vi "Set Colour.vi"(0 "Quick-GUI-Update in":refnum<class "Quick-GUI-Update.lvclass">, 2 "Label":string, 7 "Inner Color":u32(colorbox)=13816530, 9 "Outer Color":u32(colorbox)=13816530) -> (4 "Quick-GUI-Update out":refnum<class "Quick-GUI-Update.lvclass">)   [LabVIEW 2020, in "Quick-GUI-Update.lvclass"]
uses:
  Quick-GUI-Update.lvclass
  Quick-GUI-Update.lvclass/Quick-GUI-Update.ctl
  Ctrl Reference's/Ctrl Reference's.lvclass
panel:
  out "source":string
  out "code":i32
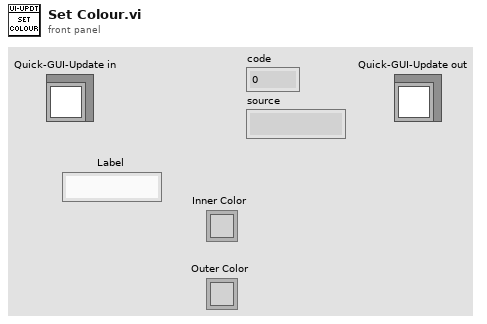
[diagram p1: front panel]
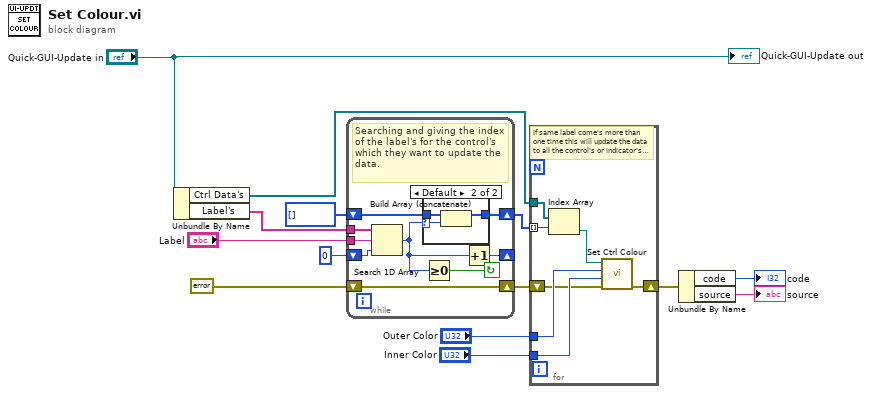
[diagram p0: block diagram]
diagram:
  n1 = Unbundle By Name("Quick-GUI-Update in") -> ("Ctrl Data's"=w13:refnum<class "Ctrl Reference's.lvclass">[], "Label's"=w10:string[])
  n2 = while {
    shift-right: [w17] -> _
    shift-left: 0 ("Start Index (0)") -> [w23]
    shift-right: [w21] -> w4
    shift-left: i32[] [] ("Initial Elements") -> [w22]
    tunnel: "Label" -> [w20]
    shift-right: [w16] -> w3
    shift-left: errorcluster {"status"=FALSE, "code"=0, "source"=""} ("error in (no error)") -> [w16]
    tunnel: w10 -> [w15]
    stop <- w18 continue-if-true
    # "Searching and giving the index of the label's for the control's which they want to update the data."
    n3 = Search 1D Array(1D array=w15, element=w20, start index (0)=w23) -> (index of element=w19:i32)
    n4 = case shown="Default" w19 {
      selector: w19 -> [_ w27]
      tunnel: w22 -> [w24 w26]
      tunnel: [w24 w25] -> w21
      frame -1 {
      }
      frame Default {
        n5 = Build Array (concatenate)(w26, w27) -> (w25:i32[])
      }
    }
    n6 = Greater Or Equal To 0?(x=w19) -> (x >= 0?=w18:bool)
    n7 = Increment(x=w19) -> (x+1=w17:i32)
  }
  n8 = for {
    shift-right: [w28] -> w9
    shift-left: w3 -> [w29]
    tunnel: w13 -> [w34]
    tunnel: w4 -> [w33] mode=indexing
    tunnel: "Outer Color" -> [w31]
    tunnel: "Inner Color" -> [w30]
    # "If same label come's more than one time this will update the data to all the control's or indicator's which contain's that label."
    n9 = Index Array(array=w34, index=w33) -> (element=w32:refnum<class "Ctrl Reference's.lvclass">)
    n10 = call "Set Ctrl Colour.vi"("error in (no error)"=w29, "Inner Color"=w30, "Outer Color"=w31, "Ctrl Reference's in"=w32) -> ("error out"=w28:errorcluster)  [unwired: 6 in, 1 out]
  }
  n11 = Unbundle By Name(w9) -> ("code"=→"code":i32, "source"=→"source":string)
  "Quick-GUI-Update out" <- "Quick-GUI-Update in"
